vi "deviceAnalysisTest_ReadTDMS.vi"() -> ()   [LabVIEW 2017]
uses:
  <vilib>/addons/InsightCM/MessageBus/Base/controls/AlarmRuleEntry.ctl
  <vilib>/addons/InsightCM/Devices/Shared/DataAccessors/controls/channelType_StatusLookup.ctl
  <vilib>/addons/InsightCM/MessageBus/Base/KeyValuePairs.ctl
  <vilib>/addons/InsightCM/MessageBus/Base/ConfigurableMetric.ctl
  <vilib>/addons/InsightCM/Utilities/ChannelStatus/controls/status.ctl
  <vilib>/addons/InsightCM/Utilities/ChannelStatus/controls/statusState.ctl
  <vilib>/addons/InsightCM/Devices/Shared/ConfigurationParsing/controls/filePaths.ctl
panel:
  in  "Tab Control":T1(tab)
  in  "Root Directory":path=path "C:/Users/Administrator/Desktop/testDevice files/testIntegrationCutoff"
  in  "Configuration Files":T2={"AlarmRules"=path "AlarmRules.json", "MetricCfg"=path "MetricConfigs.json", "HierarchyNode"=path "Hierarchy.json", "DeviceModel"=path "DeviceModel.json"}
  in  "file path":path
  out "Waveform Graph":waveform(dbl)[](graph)
  out "Waveform Graph 2":waveform(sgl)[](graph)
  out "FeatureLookup":variant
  in  "stop":bool
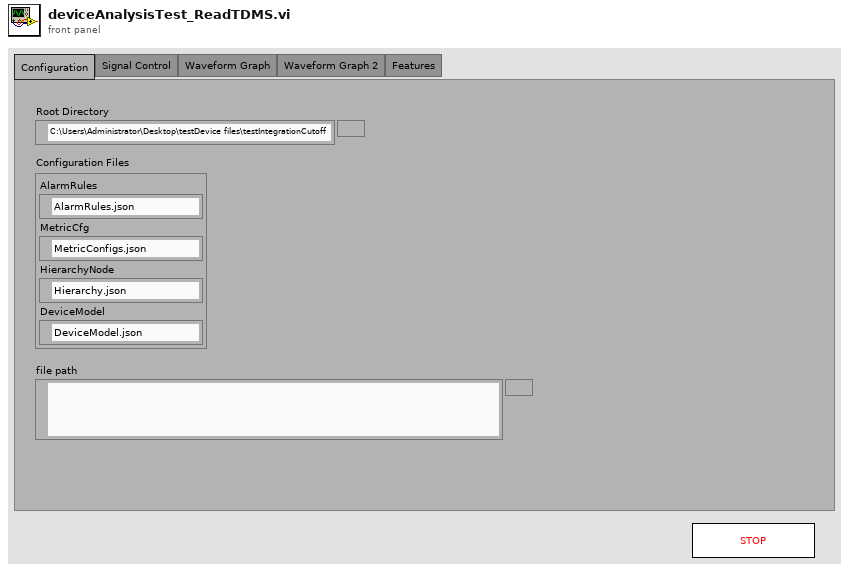
[diagram p1: front panel]
types:
  T1 = enum32{"Configuration", "Signal Control", "Waveform Graph", "Waveform Graph 2", "Features"}
  T2 = typedef "ConfigurationParsing.lvlib/filePaths.ctl" = cluster{"AlarmRules":path, "MetricCfg":path, "HierarchyNode":path, "DeviceModel":path}
  T3 = typedef "ChannelStatus.lvlib/statusState.ctl" = cluster{"channelAlias":string, "current":T4, "previous":T4, "changed":bool}
  T4 = typedef "ChannelStatus.lvlib/status.ctl" = enum16{"init", "ok", "open", "short", "outOfRange"}
  T5 = typedef "ConfigurableMetric.ctl" = cluster{"Id":i32, "MetricType":string, "Name":string, "Locked":bool, "Properties":T6}
  T6 = typedef "KeyValuePairs.ctl" = cluster{"Key":string, "Value":string}[]
  T7 = typedef "AlarmRuleEntry.ctl" = cluster{"Id":i32, "State":string, "Path":string, "Message":string, "DeviceOnly":bool, "Configuration":cluster{"Condition":string, "SetPoint":string, "Type":string, "Hysteresis":dbl, "OnDelaySeconds":dbl, "OffDelaySeconds":dbl}, "Severity":i32}
  T8 = typedef "ConfigurationParsing.lvlib/DeviceConfigData.ctl" = cluster{"Device Info":T9, "AcquisitionProperties":variant, "Channels":variant[], "StreamingProperties":variant, "DeviceSystemProperties":variant}
  T9 = typedef "ConfigurationParsing.lvlib/deviceInfo.ctl" = cluster{"Config Version":string, "DeviceID":string}
  T10 = typedef "DeviceModel.ctl" = cluster{"AssetModel":T11, "SoftwareModel":T12}
  T11 = typedef "AssetModel.ctl" = cluster{"Id":i32, "PhysicalName":string, "LogicalName":string, "PluginCodename":string, "FirmwareInfo":string, "HardwareConfig":string, "SoftwareConfigId":i32, "HierarchyNodeId":i32}
  T12 = typedef "SoftwareModel.ctl" = cluster{"Id":i32, "DeviceAssetModelId":i32, "Version":string, "Config":string, "DeviceProperties":T6, "Channels":T13[]}
  T13 = typedef "BlueRidgeChannel.ctl" = cluster{"Id":i32, "ChannelId":string, "Name":string, "ChannelCategory":string, "ChannelType":string, "ChannelTypeList":string, "HierarchyNodeId":i32, "Enabled":bool, "Properties":T6, "MetricConfigurations":T14[]}
  T14 = typedef "MetricConfiguration.ctl" = cluster{"Id":i32, "ChannelCategory":string, "MeasurementType":string, "Metrics":T15[]}
  T15 = typedef "MetricInstance.ctl" = cluster{"Id":i32, "Codename":string, "DisplayName":string, "Unit":string, "PublishToHistorian":bool, "Unscaled":bool, "Locked":bool, "TagPath":string, "Properties":T6}
  T16 = cluster{"AlarmRules":variant, "MetricCfg":variant, "HierarchyNode":variant, "DeviceConfig":T8, "DeviceModel":T10}
  T17 = typedef "AnalysisDevice.ctl" = cluster{"Device Id":string, "Dynamic Channels":T18[], "Static Channels":T26[]}
  T18 = typedef "AnalysisDynamicChannel.ctl" = cluster{"ChannelName":string, "Sensor Type":T19, "Conversion Op":T20, "Features":T21[], "Data":waveform(sgl), "Speed":sgl, "SP Index":i32, "Properties":variant, "Data Valid":bool, "Calc Measurement Type":T25}
  T19 = typedef "AnalysisSensorType.ctl" = enum16{"Accelerometer", "Velocity", "Displacement", "Tachometer", "Tempertature ", "dynamicVoltage", "Voltage", "Current", "Microphone", "Resistance", "Digital Input", "<Unknown>"}
  T20 = typedef "AnalysisConversionOp.ctl" = enum16{"none", "singleInt", "doubleInt", "singleDiff", "doubleDiff"}
  T21 = typedef "AnalysisFeature.ctl" = cluster{"Type":i32, "Code Name":string, "Unit":string, "Display Name":string, "Value":sgl, "Start":dbl, "Stop":dbl, "Band Domain":T22, "Band Calc":T23, "Amplitude Scale":T24, "Tag Path":string}
  T22 = typedef "AnalysisBandDomain.ctl" = enum16{"Frequency", "CPM", "Orders"}
  T23 = typedef "AnalysisBandCalculation.ctl" = enum16{"Total", "Max", "Phase"}
  T24 = typedef "AnalysisBandAmplitudeScale.ctl" = enum16{"rms", "peak", "pk-pk", "phase", "<none>"}
  T25 = typedef "AnalysisCalculatedMeasurementType.ctl" = enum16{"acceleration", "velocity", "displacement", "tachometer", "speed", "temperature", "voltage", "current", "resistance", "digitalInput", "<Unknown>"}
  T26 = typedef "AnalysisStaticChannel.ctl" = cluster{"ChannelName":string, "Sensor Type":T19, "Features":T21[], "Properties":variant, "Data Valid":bool, "Calc Measurement Type":T25, "Acquisition Timestamp":timestamp}
  T27 = typedef "AnalysisState.ctl" = cluster{"Properties":cluster{"File Properties":variant, "Static Properties":variant, "Waveform Properties":variant}, "Properties Initialized?":bool, "Device":T17, "Speed Profiles":T28[]}
  T28 = typedef "AnalysisSpeedProfile.ctl" = cluster{"t0":dbl, "pulse positions":sgl[], "speed":dbl}
  T29 = typedef "AnalysisBOP.lvlib/AnalysisGroups.ctl" = cluster{"StaticChannels":T30[], "TachVibrationGroups":T32[]}
  T30 = typedef "AnalysisBOP.lvlib/GeneralStaticChanAnalysisCfg.ctl" = cluster{"Wfm Index":i32, "ChannelName":string, "ChannelID":string, "bounds":T31, "TagPath":string, "Triggerable":bool}
  T31 = typedef "ChannelStatus.lvlib/outOfRangeBounds.ctl" = cluster{"maximum":dbl, "minimum":dbl}
  T32 = typedef "AnalysisBOP.lvlib/TachVibrationGroupCfg.ctl" = cluster{"TachometerChanAnalysisConfig":T33, "AnalysisChannels":T34[]}
  T33 = typedef "AnalysisBOP.lvlib/TachometerChanAnalysisCfg.ctl" = cluster{"Wfm Index":i32, "ChannelName":string, "ChannelID":string, "PulsesPerRevolution":sgl, "TachometerThreshold":sgl, "TachometerSlope":string, "TachometerHysteresis":sgl, "sampleRate":dbl, "tachometerType":string, "Analysis Wfm Index":i32}
  T34 = typedef "AnalysisBOP.lvlib/VibrationChanAnalysisCfg.ctl" = cluster{"Wfm Index":i32, "ChannelName":string, "ChannelID":string, "speedRatio":dbl, "MeasurementType":string}
  T35 = typedef "channelType_StatusLookup.ctl" = enum16{"Static", "Dynamic"}
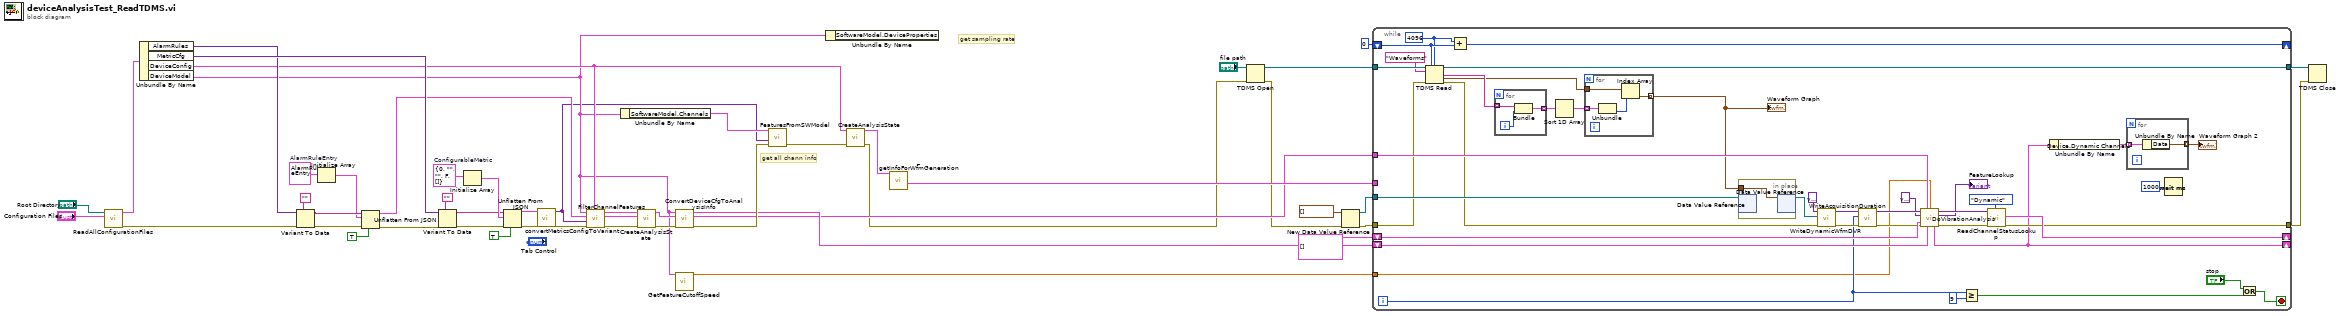
[diagram p0: block diagram]
diagram:
  w19 = T5 {"Id"=0, "MetricType"="", "Name"="", "Locked"=FALSE, "Properties"=[]}  # ConfigurableMetric
  w34 = T7 {"Id"=0, "State"="", "Path"="", "Message"="", "DeviceOnly"=FALSE, "Configuration"={"Condition"="", "SetPoint"="", "Type"="", "Hysteresis"=0.0, "OnDelaySeconds"=0.0, "OffDelaySeconds"=0.0}, "Severity"=0}  # AlarmRuleEntry
  # "get sampling rate"
  # "get all chann info"
  n1 = call <vilib>:"ReadAllConfigurationFiles.vi"("Configuration Files"="Configuration Files", "Root Directory"="Root Directory") -> ("error out"=w16:errorcluster, "Configuration"=w46:T16)  [unwired: 6 in, 2 out]
  n2 = Unbundle By Name(w46) -> ("AlarmRules"=w31:variant, "MetricCfg"=w40:variant, "DeviceConfig"=w21:T8, "DeviceModel"=w4:T10)
  n3 = Variant To Data(error in=w16, type="", Variant=w31) -> (data=w35:string, error out=w37:errorcluster)
  n4 = Initialize Array(w34) -> (w33:T7[])  [unwired: 1 in]
  n5 = Unflatten From JSON(JSON string=w35, type and defaults=w33, default null elements? (F)=TRUE, error in (no error)=w37) -> (value=w22:T7[], error out=w32:errorcluster)  [unwired: 3 in]
  n6 = Variant To Data(error in=w32, type="", Variant=w40) -> (data=w41:string, error out=w44:errorcluster)
  n7 = Initialize Array(w19) -> (w42:T5[])  [unwired: 1 in]
  n8 = Unflatten From JSON(JSON string=w41, type and defaults=w42, default null elements? (F)=TRUE, error in (no error)=w44) -> (value=w39:T5[], error out=w30:errorcluster)  [unwired: 3 in]
  n9 = call <vilib>:"convertMetricsConfigToVariant.vi"("error in (no error)"=w30, "MetricInstanceConfigs"=w39) -> ("error out"=w47:errorcluster, "metricInstanceConfig"=w1:variant)  [unwired: 8 in]
  n10 = call <vilib>:"FilterChannelFeatures.vi"("DeviceConfig"=w21, "error in (no error)"=w47, "Metric Lookup"=w1, "AlarmRules"=w22, "DeviceModel"=w4) -> ("error out"=w50:errorcluster, "Device"=w48:T17, "DeviceConfig Out"=w49:T8)  [unwired: 3 in, 1 out]
  n11 = Unbundle By Name(w4) -> ("SoftwareModel.Channels"=w20:T13[])
  n12 = call <vilib>:"CreateAnalysisState.vi"("error in (no error)"=w50, "Device"=w48, "DeviceConfig"=w49) -> ("error out"=w18:errorcluster, "Analysis State"=w15:T27)  [unwired: 7 in]
  n13 = call <vilib>:"GetFeatureCutoffSpeed.vi"("DeviceModel"=w4) -> ("featureCutoffSpeed"=w3:dbl)  [unwired: 10 in]
  n14 = call <vilib>:"ConvertDeviceCfgToAnalysisInfo.vi"("error in (no error)"=w18, "Analysis State"=w15, "DeviceModel"=w4) -> ("error out"=w17:errorcluster, "AnalysisGroups"=w13:T29, "Analysis State out"=w14:T27)  [unwired: 5 in, 1 out]
  n15 = call <vilib>:"FeaturesFromSWModel.vi"("error in (no error)"=w17, "Band Cache"=w1, "Channels"=w20) -> ("error out"=w2:errorcluster)  [unwired: 7 in, 1 out]
  n16 = Unbundle By Name(w4) -> ()  [unwired: 1 out]
  n17 = call <vilib>:"CreateAnalysisState.vi"("error in (no error)"=w2, "DeviceConfig"=w21) -> ("error out"=w11:errorcluster, "Analysis State"=w23:T27)  [unwired: 8 in]
  n18 = call <vilib>:"_getInfoForWfmGeneration.vi"("Analysis State"=w23) -> ("wfm info"=w24:cluster{i32, "variant":variant}[])  [unwired: 9 in, 1 out]
  n19 = TDMS Open(8:w11, 11:"file path") -> (0:w10:errorcluster, 3:w9:refnum<k34>)  [unwired: 5 in]
  n20 = New Data Value Reference(data value=waveform(sgl)[] [] ("wfmData"), error in=w10) -> (data value reference=w26:refnum<data-value>, error out=w27:errorcluster)
  n21 = while {
    tunnel: w27 -> [w68]
    shift-right: [w90] -> _
    shift-left: T3[] [] ("channel status") -> [w89]
    tunnel: w26 -> [w84]
    tunnel: [w76] -> w8
    tunnel: w24 -> [_]
    shift-right: [w70] -> _
    shift-left: w14 -> [w72]
    tunnel: w13 -> [w71]
    tunnel: w9 -> [w69]
    tunnel: [w66] -> w7
    shift-right: [w60] -> _
    shift-left: 0 -> [w62]
    tunnel: w3 -> [w51]
    i -> [w59]
    stop <- w63 stop-if-true
    w61 = i64 4096 ("count (-1: all)")
    n22 = TDMS Read(0:w69, 1:w62, 2:w61, 5:"Waveforms" ("group name in"), 11:w68) -> (4:w66:refnum<k34>, 8:w56:string[], 10:w53:waveform(dbl)[], 15:w67:errorcluster)  [unwired: 3 in, 2 out]
    n23 = Add(x=w61, y=w62) -> (x+y=w60:i64)
    n24 = for {
      tunnel: w56 -> [w97] mode=indexing
      tunnel: [w96] -> w55 mode=indexing
      i -> [w95]
      n25 = Bundle(w97, w95) -> (w96:cluster{string, i32})  [unwired: 1 in]
    }
    n26 = Sort 1D Array(array=w55) -> (sorted array=w54:cluster{string, i32}[])
    n27 = for {
      tunnel: w54 -> [w93] mode=indexing
      tunnel: w53 -> [w94]
      tunnel: [w91] -> w52 mode=indexing
      n28 = Unbundle(w93) -> (w92:i32)  [unwired: 1 out]
      n29 = Index Array(array=w94, index=w92) -> (element=w91:waveform(dbl))
    }
    "Waveform Graph" <- w52
    n30 = in-place {
      in-place-border: w52 -> [w100]
      n31 = in-place-dvr #1(w84) -> ()  [unwired: 2 out]
      n32 = in-place-dvr #1(w100) -> (w83:refnum<data-value>)  [unwired: 1 out]
    }
    n33 = call <vilib>:"WriteDynamicWfmDVR.vi"("error in (no error)"=w67, "dynamic Wfm DVR"=w83, "variant"=variant) -> ("error out"=w88:errorcluster, "variant"=w87:variant)  [unwired: 7 in]
    n34 = call <vilib>:"WriteAcquisitionDuration.vi"("error in (no error)"=w88, "acquisitionDuration"=w59, "variant"=w87) -> ("error out"=w85:errorcluster, "variant"=w86:variant)  [unwired: 7 in]
    n35 = call <vilib>:"DoVibrationAnalysis.vi"("variant"=w86, "AnalysisGroups"=w71, "FeatureSpeedCutoff"=w51, "featureLookup"=variant, "channel status"=w89, "error in (no error)"=w85, "Analysis State"=w72) -> ("variant out"=w79:variant, "FeatureLookup"=→"FeatureLookup":variant, "Analysis State Out"=w70:T27, "error out"=w78:errorcluster)  [unwired: 4 in, 1 out]
    n36 = Greater Or Equal?(x=w59, y=9) -> (x >= y?=w57:bool)
    n37 = call <vilib>:"ReadChannelStatusLookup.vi"("channel type"=channelType_StatusLookup."Dynamic", "error in (no error)"=w78, "variant"=w79) -> ("error out"=w76:errorcluster, "channel status"=w90:T3[])  [unwired: 6 in, 1 out]
    n38 = Unbundle By Name(w70) -> ("Device.Dynamic Channels"=w75:T18[])
    n39 = for {
      tunnel: w75 -> [w99] mode=indexing
      tunnel: [w98] -> w74 mode=indexing
      n40 = Unbundle By Name(w99) -> ("Data"=w98:waveform(sgl))
    }
    "Waveform Graph 2" <- w74
    n41 = Wait (ms)(milliseconds to wait=u32 1000) -> ()  [unwired: 1 out]
    n42 = Or(x="stop", y=w57) -> (x .or. y?=w63:bool)
  }
  n43 = TDMS Close(8:w8, 11:w7) -> ()  [unwired: 2 out]
